vi "Get Library Class Name.vi"(11 "VI In":string) -> (0 "Found?":bool, 3 "Lib_Class name":string)   [LabVIEW 2019, in "DependencyInspector.lvlib"]
uses:
  DependencyInspector.lvlib
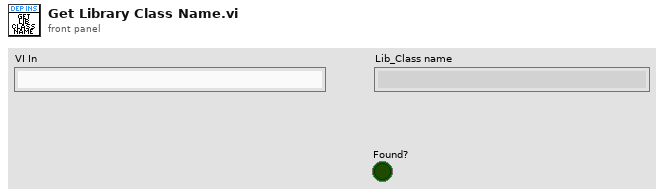
[diagram p1: front panel]
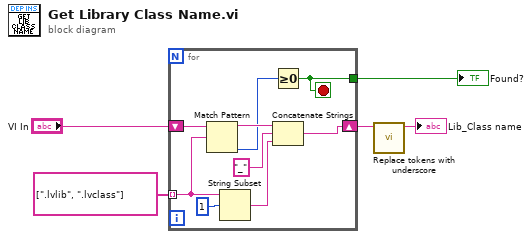
[diagram p0: block diagram]
diagram:
  n1 = for {
    tunnel: string[] [".lvlib", ".lvclass"] ("regular expression") -> [w8] mode=indexing
    shift-right: [w10] -> w2
    shift-left: "VI In" -> [w14]
    tunnel: [w11] -> w3
    stop <- w11 stop-if-true
    n2 = Match Pattern(string=w14, regular expression=w8) -> (before substring=w13:string, offset past match=w12:i32)  [unwired: 1 in, 2 out]
    n3 = String Subset(string=w8, offset (0)=1) -> (substring=w7:string)  [unwired: 1 in]
    n4 = Greater Or Equal To 0?(x=w12) -> (x >= 0?=w11:bool)
    n5 = Concatenate Strings(w13, "_", w7) -> (w10:string)
  }
  "Found?" <- w3
  n6 = call "Replace tokens with underscore.vi"("Sting"=w2) -> ("sanitized"=→"Lib_Class name":string)  [unwired: 10 in]
